vi "player-modified.vi"() -> ()   [LabVIEW 2012]
uses:
  <vilib>/Utility/error.llb/DialogType.ctl
  player_glo.vi
  musicplayer_glo.vi
  test_glo.vi
panel:
  out "playState":i32(ring) items=["wmppsUndefined", "wmppsStopped", "wmppsPaused", "wmppsPlaying", "wmppsScanForward", "wmppsScanReverse", "wmppsBuffering", "wmppsWaiting", "wmppsMediaEnded", "wmppsTransitioning", "wmppsReady", "wmppsReconnecting", "wmppsLast"]
  in  "started?":bool
  in  "WindowsMediaPlayer":refnum<k7>(container)
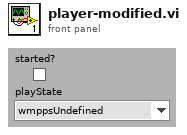
[diagram p1: front panel]
types:
  T1 = typedef "DialogType.ctl" = u16
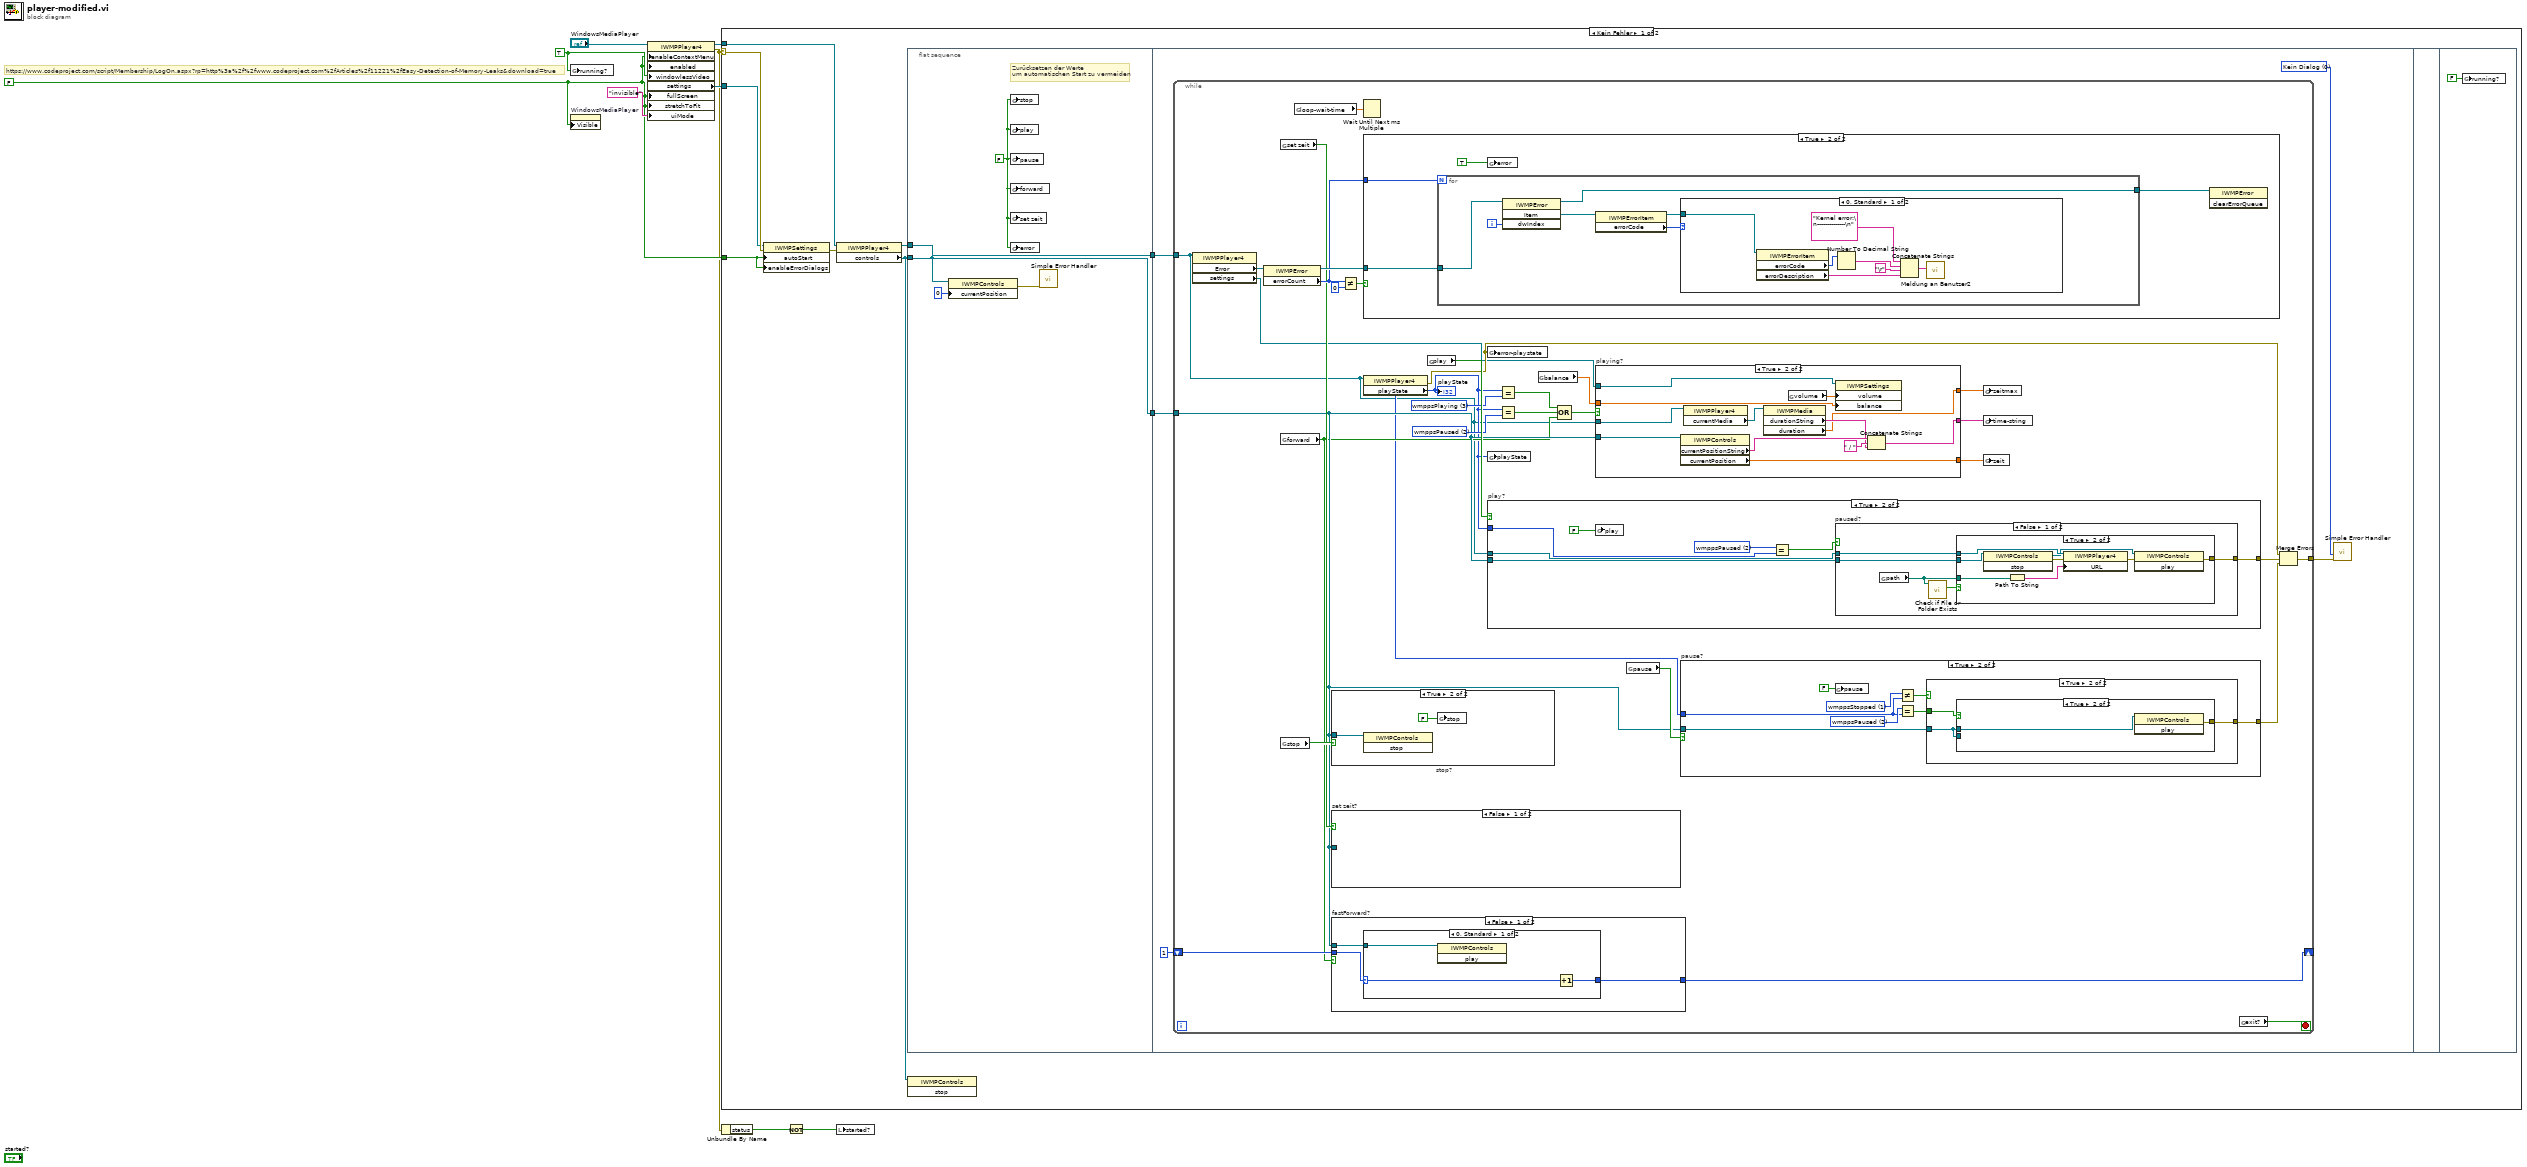
[diagram p0: block diagram]
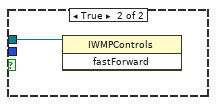
[diagram p3: hidden frame]
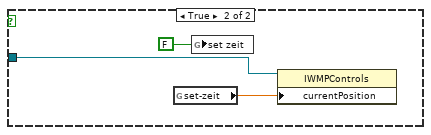
[diagram p4: hidden frame]
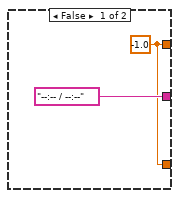
[diagram p5: hidden frame]
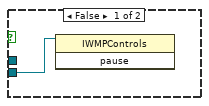
[diagram p8: hidden frame]
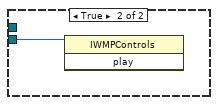
[diagram p12: hidden frame]
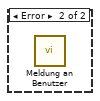
[diagram p15: hidden frame]
diagram:
  w9 = TRUE ("windowlessVideo")
  w4 = FALSE ("enableContextMenu")
  # "https://www.codeproject.com/script/Membership/LogOn.aspx?rp=http%3a%2f%2fwww.codeproject.com%2fArticles%2f11221%2fEasy-Detection-of-Memory-Leaks&download=true"
  n1 = global write "player_glo.vi" "running?"(w9) -> ()
  n2 = property on="WindowsMediaPlayer" class="AXCont"("Visible"=w4) -> ()  [unwired: 2 in, 2 out]
  n3 = property class="IWMPPlayer4"(reference="WindowsMediaPlayer", "enableContextMenu"=w4, "enabled"=w4, "windowlessVideo"=w9, "fullScreen"=w4, "stretchToFit"=w4, "uiMode"="invisible") -> (reference out=w6:refnum<k7>, error out=w1:errorcluster, "settings"=w5:refnum<k7>)  [unwired: 1 in]
  n4 = case shown="Kein Fehler" w1 {
    selector: w1 -> [w13 _]
    tunnel: w6 -> [w12 _]
    tunnel: w5 -> [w11 _]
    tunnel: w4 -> [w10 _]
    frame No Error {
      n5 = property class="IWMPSettings"(reference=w11, error in=w13, "autoStart"=w10, "enableErrorDialogs"=w10) -> (error out=w18:errorcluster)  [unwired: 1 out]
      n6 = property class="IWMPPlayer4"(reference=w12, error in=w18) -> (reference out=w17:refnum<k7>, "controls"=w16:refnum<k7>)  [unwired: 1 out]
      n7 = flat-sequence {
        tunnel: w16 -> [w21]
        tunnel: w17 -> [w23]
        tunnel: [w23] -> w15
        tunnel: [w21] -> w14
        tunnel: w15 -> [w27]
        tunnel: w14 -> [w28]
        frame #0 {
          w22 = FALSE
          # "Zurücksetzen der Werte\num automatischen Start zu vermeiden"
          n8 = property class="IWMPControls"(reference=w21, "currentPosition"=0) -> (error out=w19:errorcluster)  [unwired: 1 in, 1 out]
          n9 = global write "player_glo.vi" "stop"(w22) -> ()
          n10 = global write "player_glo.vi" "play"(w22) -> ()
          n11 = global write "player_glo.vi" "pause"(w22) -> ()
          n12 = global write "player_glo.vi" "forward"(w22) -> ()
          n13 = global write "player_glo.vi" "set zeit"(w22) -> ()
          n14 = global write "player_glo.vi" "error"(w22) -> ()
          n15 = call <vilib>:"Simple Error Handler.vi"("error in (no error)"=w19) -> ()  [unwired: 4 in, 5 out]
        }
        frame #1 {
          w24 = T1 0 items=["Kein Dialog", "OK-Meldung", "Dialog zum Fortsetzen oder Anhalten", "OK-Meldung + Warnungen", "Weiter/Stopp + Warnung"] ("type of dialog (OK msg:1)")
          n16 = while {
            tunnel: w27 -> [w31]
            tunnel: w28 -> [w40]
            shift-right: [w41] -> _
            shift-left: 1 -> [w42]
            tunnel: [w37] -> w25
            stop <- w55 stop-if-true
            w47 = 2 items=["wmppsUndefined", "wmppsStopped", "wmppsPaused", "wmppsPlaying", "wmppsScanForward", "wmppsScanReverse", "wmppsBuffering", "wmppsWaiting", "wmppsMediaEnded", "wmppsTransitioning", "wmppsReady", "wmppsReconnecting", "wmppsLast"] ("playState")
            w51 = 3 items=["wmppsUndefined", "wmppsStopped", "wmppsPaused", "wmppsPlaying", "wmppsScanForward", "wmppsScanReverse", "wmppsBuffering", "wmppsWaiting", "wmppsMediaEnded", "wmppsTransitioning", "wmppsReady", "wmppsReconnecting", "wmppsLast"] ("playState")
            n17 = property class="IWMPPlayer4"(reference=w31) -> ("Error"=w30:refnum<k7>, "settings"=w29:refnum<k7>)  [unwired: 1 in, 2 out]
            n18 = property class="IWMPError"(reference=w30) -> (reference out=w58:refnum<k7>, "errorCount"=w56:i32)  [unwired: 1 in, 1 out]
            n19 = global read "player_glo.vi" "set zeit"() -> (w43:bool)
            n20 = global read "player_glo.vi" "forward"() -> (w36:bool)
            n21 = global read "player_glo.vi" "stop"() -> (w53:bool)
            n22 = global read "player_glo.vi" "loop-wait-time"() -> (w48:dbl)
            n23 = case "stop?" shown="True" w53 {
              tunnel: w40 -> [_ w99]
              frame False {
              }
              frame True {
                n24 = invoke class="IWMPControls" method="stop"(reference=w99) -> ()  [unwired: 2 in, 3 out]
                n25 = global write "player_glo.vi" "stop"(FALSE) -> ()
              }
            }
            n26 = case "set zeit?" shown="False" w43 {
              tunnel: w40 -> [_ w70]
              frame False {
              }
              frame True {
                n27 = global read "player_glo.vi" "set-zeit"() -> (w69:dbl)
                n28 = global write "player_glo.vi" "set zeit"(FALSE) -> ()
                n29 = property class="IWMPControls"(reference=w70, "currentPosition"=w69) -> ()  [unwired: 1 in, 2 out]
              }
            }
            n30 = case "fastForward?" shown="False" w36 {
              tunnel: w40 -> [w62 w67]
              tunnel: w42 -> [w61 _]
              tunnel: [w60 _] -> w41
              frame False {
                n31 = case shown="0, Standard" w61 {
                  selector: w61 -> [w65 w66]
                  tunnel: w62 -> [w63 _]
                  tunnel: [w64 w66] -> w60
                  frame 0, Default {
                    n32 = invoke class="IWMPControls" method="play"(reference=w63) -> ()  [unwired: 2 in, 3 out]
                    n33 = Increment(x=w65) -> (x+1=w64:i32)
                  }
                  frame 1 {
                  }
                }
              }
              frame True {
                n34 = invoke class="IWMPControls" method="fastForward"(reference=w67) -> ()  [unwired: 2 in, 3 out]
              }
            }
            n35 = Not Equal?(x=w56, y=0) -> (x != y?=w59:bool)
            n36 = Wait Until Next ms Multiple(millisecond multiple=w48) -> ()  [unwired: 1 out]
            n37 = case shown="True" w59 {
              tunnel: w58 -> [_ w125]
              tunnel: w56 -> [_ w124]
              frame False {
              }
              frame True {
                n38 = for {
                  N: w124 -> [_]
                  tunnel: w125 -> [w131]
                  tunnel: [w126] -> w122
                  i -> [w130]
                  n39 = invoke class="IWMPError" method="Item"(reference=w131, "dwIndex"=w130) -> (reference out=w126:refnum<k7>, "Item"=w129:refnum<k7>)  [unwired: 2 in, 2 out]
                  n40 = property class="IWMPErrorItem"(reference=w129) -> (reference out=w127:refnum<k7>, "errorCode"=w128:i32)  [unwired: 1 in, 1 out]
                  n41 = case shown="0, Standard" w128 {
                    tunnel: w127 -> [w136 _]
                    frame 0, Default {
                      n42 = property class="IWMPErrorItem"(reference=w136) -> ("errorCode"=w135:i32, "errorDescription"=w132:string)  [unwired: 1 in, 2 out]
                      n43 = Number To Decimal String(number=w135) -> (decimal integer string=w134:string)  [unwired: 1 in]
                      n44 = Concatenate Strings("Kernel error:\n--------------\n" ("String"), w134, "\r", w132) -> (w138:string)
                      n45 = call "Meldung an Benutzer2"("Message"=w138) -> ()  [unwired: 9 in, 2 out]
                    }
                    frame -1072885353 {
                      # "fehler mit file"
                    }
                  }
                }
                n46 = global write "player_glo.vi" "error"(TRUE ("error")) -> ()
                n47 = invoke class="IWMPError" method="clearErrorQueue"(reference=w122) -> ()  [unwired: 2 in, 3 out]
              }
            }
            n48 = property class="IWMPPlayer4"(reference=w31) -> (error out=w34:errorcluster, "playState"=w32:i32)  [unwired: 1 in, 1 out]
            "playState" <- w32
            n49 = global read "player_glo.vi" "play"() -> (w54:bool)
            n50 = global write "test_glo.vi" "error-playstate"(w34) -> ()
            n51 = global write "player_glo.vi" "playState"(w32) -> ()
            n52 = case "play?" shown="True" w54 {
              tunnel: w40 -> [_ w106]
              tunnel: w31 -> [_ w107]
              tunnel: w32 -> [_ w103]
              tunnel: [_ w101] -> w39
              frame False {
              }
              frame True {
                w105 = 2 items=["wmppsUndefined", "wmppsStopped", "wmppsPaused", "wmppsPlaying", "wmppsScanForward", "wmppsScanReverse", "wmppsBuffering", "wmppsWaiting", "wmppsMediaEnded", "wmppsTransitioning", "wmppsReady", "wmppsReconnecting", "wmppsLast"] ("playState")
                n53 = global write "player_glo.vi" "play"(FALSE ("play")) -> ()
                n54 = Equal?(x=w105, y=w103) -> (x = y?=w104:bool)
                n55 = case "paused?" shown="False" w104 {
                  tunnel: w107 -> [w111 _]
                  tunnel: w106 -> [w109 w121]
                  tunnel: [w108 _] -> w101
                  frame False {
                    n56 = global read "player_glo.vi" "path"() -> (w110:path)
                    n57 = call <vilib>:"Check if File or Folder Exists.vi"("path"=w110) -> ("file or folder exists?"=w112:bool)  [unwired: 8 in, 2 out]
                    n58 = case shown="True" w112 {
                      tunnel: w111 -> [_ w118]
                      tunnel: w110 -> [_ w120]
                      tunnel: w109 -> [_ w117]
                      tunnel: [_ w115] -> w108
                      frame False {
                      }
                      frame True {
                        n59 = invoke class="IWMPControls" method="stop"(reference=w117) -> (reference out=w116:refnum<k7>, error out=w113:errorcluster)  [unwired: 2 in, 1 out]
                        n60 = Path To String(path=w120) -> (string=w119:string)
                        n61 = property class="IWMPPlayer4"(reference=w118, error in=w113, "URL"=w119) -> (error out=w114:errorcluster)  [unwired: 1 out]
                        n62 = invoke class="IWMPControls" method="play"(reference=w116, error in=w114) -> (error out=w115:errorcluster)  [unwired: 1 in, 2 out]
                      }
                    }
                  }
                  frame True {
                    n63 = invoke class="IWMPControls" method="play"(reference=w121) -> ()  [unwired: 2 in, 3 out]
                  }
                }
              }
            }
            n64 = Equal?(x=w32, y=w51) -> (x = y?=w50:bool)
            n65 = Equal?(x=w32, y=w47) -> (x = y?=w35:bool)
            n66 = global read "player_glo.vi" "balance"() -> (w33:dbl)
            n67 = Compound Arithmetic op=OR(w50, w35, w36) -> (w49:bool)
            n68 = case "playing?" shown="True" w49 {
              tunnel: w40 -> [_ w84]
              tunnel: ["--:-- / --:--" w80] -> w46
              tunnel: [w71 w79] -> w45
              tunnel: [w71 w78] -> w44
              tunnel: w33 -> [_ w75]
              tunnel: w31 -> [_ w73]
              tunnel: w29 -> [_ w74]
              frame False {
                w71 = -1.0 ("currentPosition")
              }
              frame True {
                n69 = property class="IWMPControls"(reference=w84) -> ("currentPositionString"=w83:string, "currentPosition"=w79:dbl)  [unwired: 1 in, 2 out]
                n70 = property class="IWMPPlayer4"(reference=w73) -> ("currentMedia"=w77:refnum<k7>)  [unwired: 1 in, 2 out]
                n71 = property class="IWMPMedia"(reference=w77) -> ("durationString"=w81:string, "duration"=w78:dbl)  [unwired: 1 in, 2 out]
                n72 = global read "player_glo.vi" "volume"() -> (w76:dbl)
                n73 = property class="IWMPSettings"(reference=w74, "volume"=w76, "balance"=w75) -> ()  [unwired: 1 in, 2 out]
                n74 = Concatenate Strings(w83, " / ", w81) -> (w80:string)
              }
            }
            n75 = global read "player_glo.vi" "pause"() -> (w52:bool)
            n76 = case "pause?" shown="True" w52 {
              tunnel: w40 -> [_ w90]
              tunnel: w32 -> [_ w88]
              tunnel: [_ w85] -> w38
              frame False {
              }
              frame True {
                w89 = 1 items=["wmppsUndefined", "wmppsStopped", "wmppsPaused", "wmppsPlaying", "wmppsScanForward", "wmppsScanReverse", "wmppsBuffering", "wmppsWaiting", "wmppsMediaEnded", "wmppsTransitioning", "wmppsReady", "wmppsReconnecting", "wmppsLast"] ("playState")
                w91 = 2 items=["wmppsUndefined", "wmppsStopped", "wmppsPaused", "wmppsPlaying", "wmppsScanForward", "wmppsScanReverse", "wmppsBuffering", "wmppsWaiting", "wmppsMediaEnded", "wmppsTransitioning", "wmppsReady", "wmppsReconnecting", "wmppsLast"] ("playState")
                n77 = global write "player_glo.vi" "pause"(FALSE ("pause")) -> ()
                n78 = Not Equal?(x=w89, y=w88) -> (x != y?=w86:bool)
                n79 = Equal?(x=w91, y=w88) -> (x = y?=w87:bool)
                n80 = case shown="True" w86 {
                  tunnel: w90 -> [_ w95]
                  tunnel: w87 -> [_ w94]
                  tunnel: [_ w93] -> w85
                  frame False {
                  }
                  frame True {
                    n81 = case shown="True" w94 {
                      tunnel: w95 -> [_ w98]
                      tunnel: w95 -> [w96 _]
                      tunnel: [_ w97] -> w93
                      frame False {
                        n82 = invoke class="IWMPControls" method="pause"(reference=w96) -> ()  [unwired: 2 in, 3 out]
                      }
                      frame True {
                        n83 = invoke class="IWMPControls" method="play"(reference=w98) -> (error out=w97:errorcluster)  [unwired: 2 in, 2 out]
                      }
                    }
                  }
                }
              }
            }
            n84 = global write "player_glo.vi" "zeitmax"(w44) -> ()
            n85 = global write "player_glo.vi" "time-string"(w46) -> ()
            n86 = global write "player_glo.vi" "zeit"(w45) -> ()
            n87 = global read "musicplayer_glo.vi" "exit?"() -> (w55:bool)
            n88 = Merge Errors(w34, w39, w38) -> (w37:errorcluster)
          }
          n89 = call <vilib>:"Simple Error Handler.vi"("type of dialog (OK msg:1)"=w24, "error in (no error)"=w25) -> ()  [unwired: 3 in, 5 out]
        }
        frame #2 {
        }
        frame #3 {
          n90 = global write "player_glo.vi" "running?"(FALSE) -> ()
        }
      }
      n91 = invoke class="IWMPControls" method="stop"(reference=w16) -> ()  [unwired: 2 in, 3 out]
    }
    frame Error {
      n92 = call "Meldung an Benutzer"() -> ()  [unwired: 3 in, 9 out]
    }
  }
  n93 = Unbundle By Name(w1) -> ("status"=w3:bool)
  n94 = Not(x=w3) -> (.not. x?=w2:bool)
  n95 = local write "started?"(w2) -> ()
